vi "retrieveCategory.vi"(8 "error in (no error)":errorcluster, 10 "Category.lvclass":refnum<class "Category.lvclass">, 11 "Account History in":refnum<class "Account History.lvclass">) -> (0 "error out":errorcluster, 2 "Category out":refnum<class "Category.lvclass">, 3 "Account History out":refnum<class "Account History.lvclass">)   [LabVIEW 2018, in "Account History.lvclass"]
uses:
  Account History.lvclass
  Category/Category.lvclass
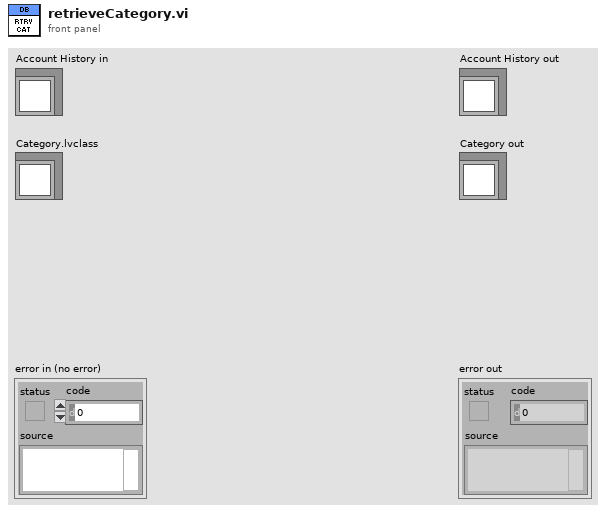
[diagram p1: front panel]
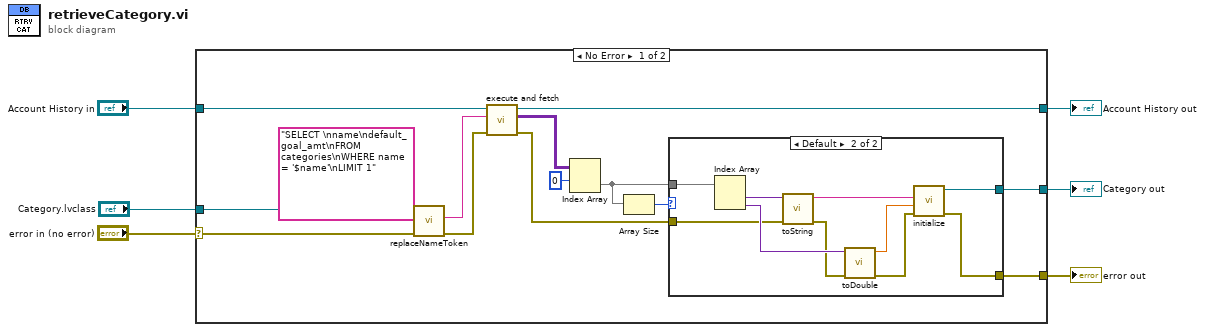
[diagram p0: block diagram]
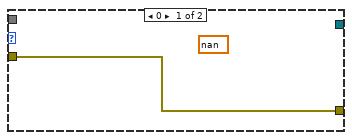
[diagram p2: hidden frame]
diagram:
  n1 = case shown="No Error" "error in (no error)" {
    selector: "error in (no error)" -> [w13 w33]
    tunnel: [w17 w33] -> w5
    tunnel: [w18 w32] -> w3
    tunnel: "Account History in" -> [w19 w32]
    tunnel: "Category.lvclass" -> [w12 _]
    tunnel: [w7 _] -> w1
    frame No Error {
      n2 = call "replaceNameToken.vi"("error in (no error)"=w13, "Query In"="SELECT \nname\ndefault_goal_amt\nFROM categories\nWHERE name = '$name'\nLIMIT 1", "Category in"=w12) -> ("error out"=w16:errorcluster, "Query Out"=w15:string)  [unwired: 6 in, 1 out]
      n3 = call "execute and fetch.vi"("error in (no error)"=w16, "SQL query"=w15, "Database in"=w19) -> ("error out"=w20:errorcluster, "recordset data"=w10:variant[][], "Database out"=w18:refnum<class "Account History.lvclass">)  [unwired: 5 in, 1 out]
      n4 = Index Array(array=w10, index (row)=0) -> (element=w9:variant[])  [unwired: 1 in]
      n5 = Array Size(array=w9) -> (size(s)=w8:i32)
      n6 = case shown="Default" w8 {
        tunnel: w20 -> [w21 w28]
        tunnel: [w21 w23] -> w17
        tunnel: w9 -> [_ w31]
        tunnel: [_ w22] -> w7
        frame 0 {
          (unwired) nan ("type")
        }
        frame Default {
          n7 = Index Array(array=w31) -> (element #1=w30:variant, element #2=w29:variant)  [unwired: 2 in]
          n8 = call "toString.vi"("error in (no error)"=w28, "Variant"=w30) -> ("error out"=w27:errorcluster, "String"=w26:string)  [unwired: 8 in]
          n9 = call "toDouble.vi"("error in (no error)"=w27, "Value"=w29) -> ("error out"=w24:errorcluster, "type"=w25:dbl)  [unwired: 8 in]
          n10 = call "initialize.vi"("error in (no error)"=w24, "Default Goal Amount"=w25, "Name"=w26) -> ("error out"=w23:errorcluster, "Category out"=w22:refnum<class "Category.lvclass">)  [unwired: 7 in]
        }
      }
    }
    frame Error {
    }
  }
  "error out" <- w5
  "Account History out" <- w3
  "Category out" <- w1
